vi "tearDown.vi"(8 "error in (no error)":errorcluster, 11 "reference in":refnum<class "Test TCP Nested Endpoint Nonforwarded Messages.lvclass">) -> (0 "error out":errorcluster, 3 "reference out":refnum<class "Test TCP Nested Endpoint Nonforwarded Messages.lvclass">)   [LabVIEW 2020, in "Test TCP Nested Endpoint Nonforwarded Messages.lvclass"]
doc: "tearDown runs after the test method has completed. Use this method to clean up any operations or references that were opened by setUp or the test method. Unit tests should be independent of other unit tests so this VI should ensure that the next test can run in a 'clean' test environment."
uses:
  Test TCP Nested Endpoint Nonforwarded Messages.lvclass
  <vilib>/ActorFramework/Message Queue/Message Queue.lvclass
  <vilib>/ActorFramework/Stop Msg/Stop Msg.lvclass
  Source/Protocols/TCP Strategy/TCP Stream Listener/TCP Stream Listener.lvclass
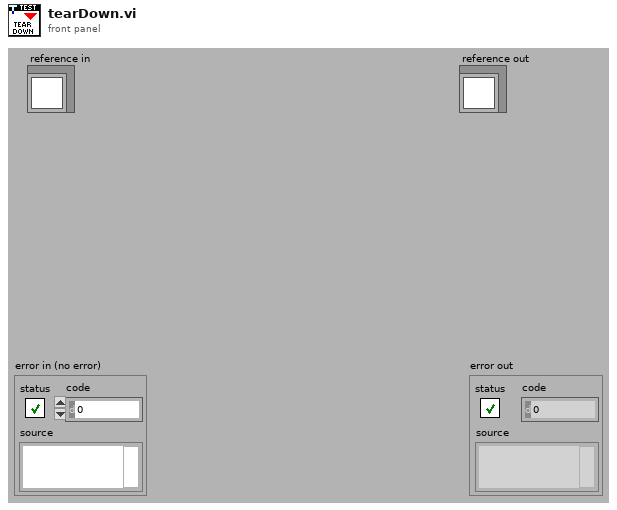
[diagram p1: front panel]
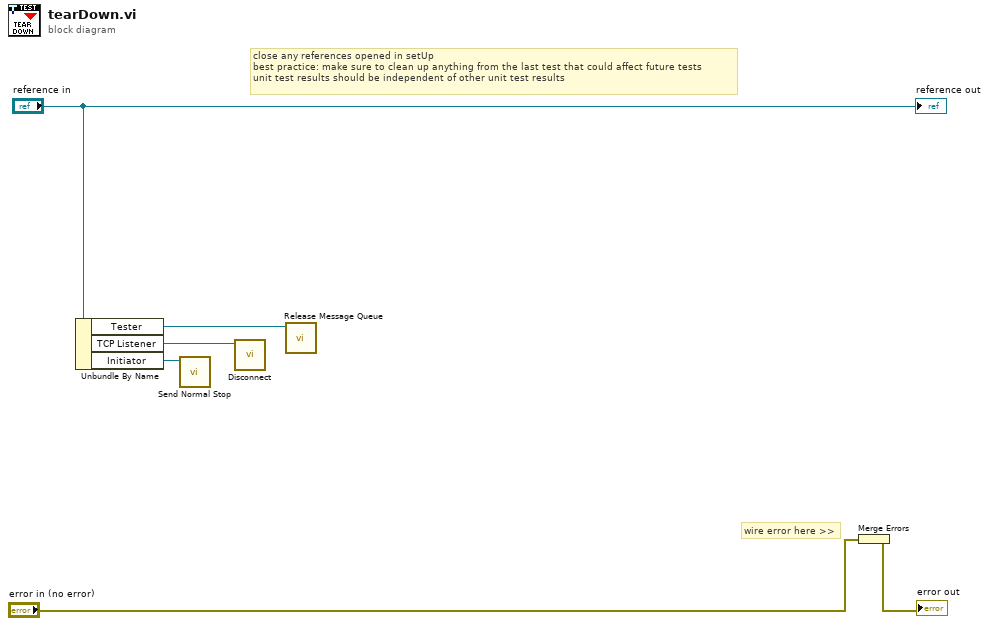
[diagram p0: block diagram]
diagram:
  # "wire error here >>"
  # "close any references opened in setUp\nbest practice: make sure to clean up anything from the last test that could affect future tests\nunit test results should be independent of other unit test results"
  n1 = Unbundle By Name("reference in") -> ("Tester"=w3:refnum<class "Message Queue.lvclass">, "TCP Listener"=w1:refnum<class "TCP Stream Listener.lvclass">, "Initiator"=w2:refnum<class "Message Enqueuer.lvclass">)
  n2 = call <vilib>:"Send Normal Stop.vi"("Message Enqueuer"=w2) -> ()  [unwired: 10 in, 1 out]
  n3 = call-dynamic "Disconnect.vi"("TCP Stream in"=w1) -> ()  [unwired: 9 in, 2 out]
  n4 = call <vilib>:"Release Message Queue.vi"("Message Queue"=w3) -> ()  [unwired: 9 in, 2 out]
  n5 = Merge Errors("error in (no error)") -> (→"error out":errorcluster)
  "reference out" <- "reference in"
